vi "Volt_to_USB.vi"() -> ()   [LabVIEW 2015]
panel:
  out "ERROR STATUS":string
  in  "Actuator 1 to 37":i32[](array[numeric])
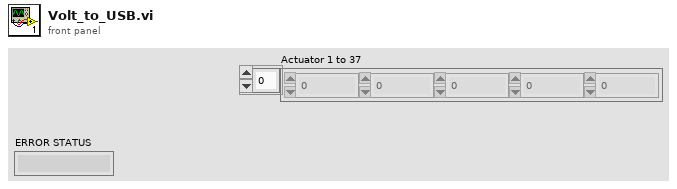
[diagram p1: front panel]
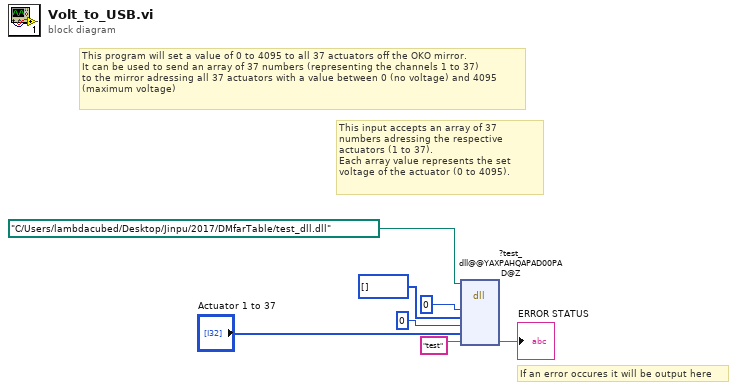
[diagram p0: block diagram]
diagram:
  # "This input accepts an array of 37 numbers adressing the respective actuators (1 to 37).\nEach array value represents the set voltage of the actuator (0 to 4095)."
  # "If an error occures it will be output here"
  # "This program will set a value of 0 to 4095 to all 37 actuators off the OKO mirror.\nIt can be used to send an array of 37 numbers (representing the channels 1 to 37) \nto the mirror adressing all 37 actuators with a value between 0 (no voltage) and 4095\n(maximum voltage)"
  n1 = dll-call lib="C:/Users/lambdacubed/Desktop/Jinpu/2017/DMfarTable/test_dll.dll" fn="?test_dll@@YAXPAHQAPAD00PAD@Z"(path in=path "C:/Users/lambdacubed/Desktop/Jinpu/2017/DMfarTable/test_dll.dll", "argc"=0, "argv"=i32[] [], "channel"=0, "voltage"="Actuator 1 to 37", "status"="test") -> ("status"=→"ERROR STATUS":string)  [unwired: 7 in, 2 out]
